vi "SiRealCenterFinder.vi"() -> ()   [LabVIEW 2019]
uses:
  <vilib>/userDefined/High Color/IMAQdx.ctl
panel:
  in  "AdjustCamera":T1={"+Y"=FALSE, "-Z"=FALSE, "Done"=FALSE, "+Z"=FALSE, "-Y"=FALSE, "-X"=FALSE, "+X"=FALSE, "MoveXYBy(mm)"=0.25, "Gcode"="", "MoveZBy(mm)"=0.1} {"MoveZBy(mm)" format="%#_13g"}
  out "CameraGcode":string
  in  "SiOnBPFiducials":path=path "C:/Users/TTUHEP/Documents/LabVIEW/Data/AssemblyIO_logs/Si2Fiducials_onBP.txt"
  out "Dev":dbl
  out "ImageCurrent":T2(plugin-control)
  out "Image2":T2(plugin-control)
  out "Image1":T2(plugin-control)
  out "Output XYZU":string
  in  "HexaboardEdges":path=path "C:/Users/TTUHEP/Documents/LabVIEW/Data/AssemblyIO_logs/PCB1_4Points.txt"
  in  "SiFiducials":path=path "C:/Users/TTUHEP/Documents/LabVIEW/Data/AssemblyIO_logs/Si2Fiducials.txt"
  in  "Component":enum16{"Baseplate", "Si", "SiOnBP", "PCB"}(ring)=enum."Si"
  in  "BasePlateEdges":path=path "C:/Users/TTUHEP/Documents/LabVIEW/Data/AssemblyIO_logs/Baseplate1CuPoints.txt"
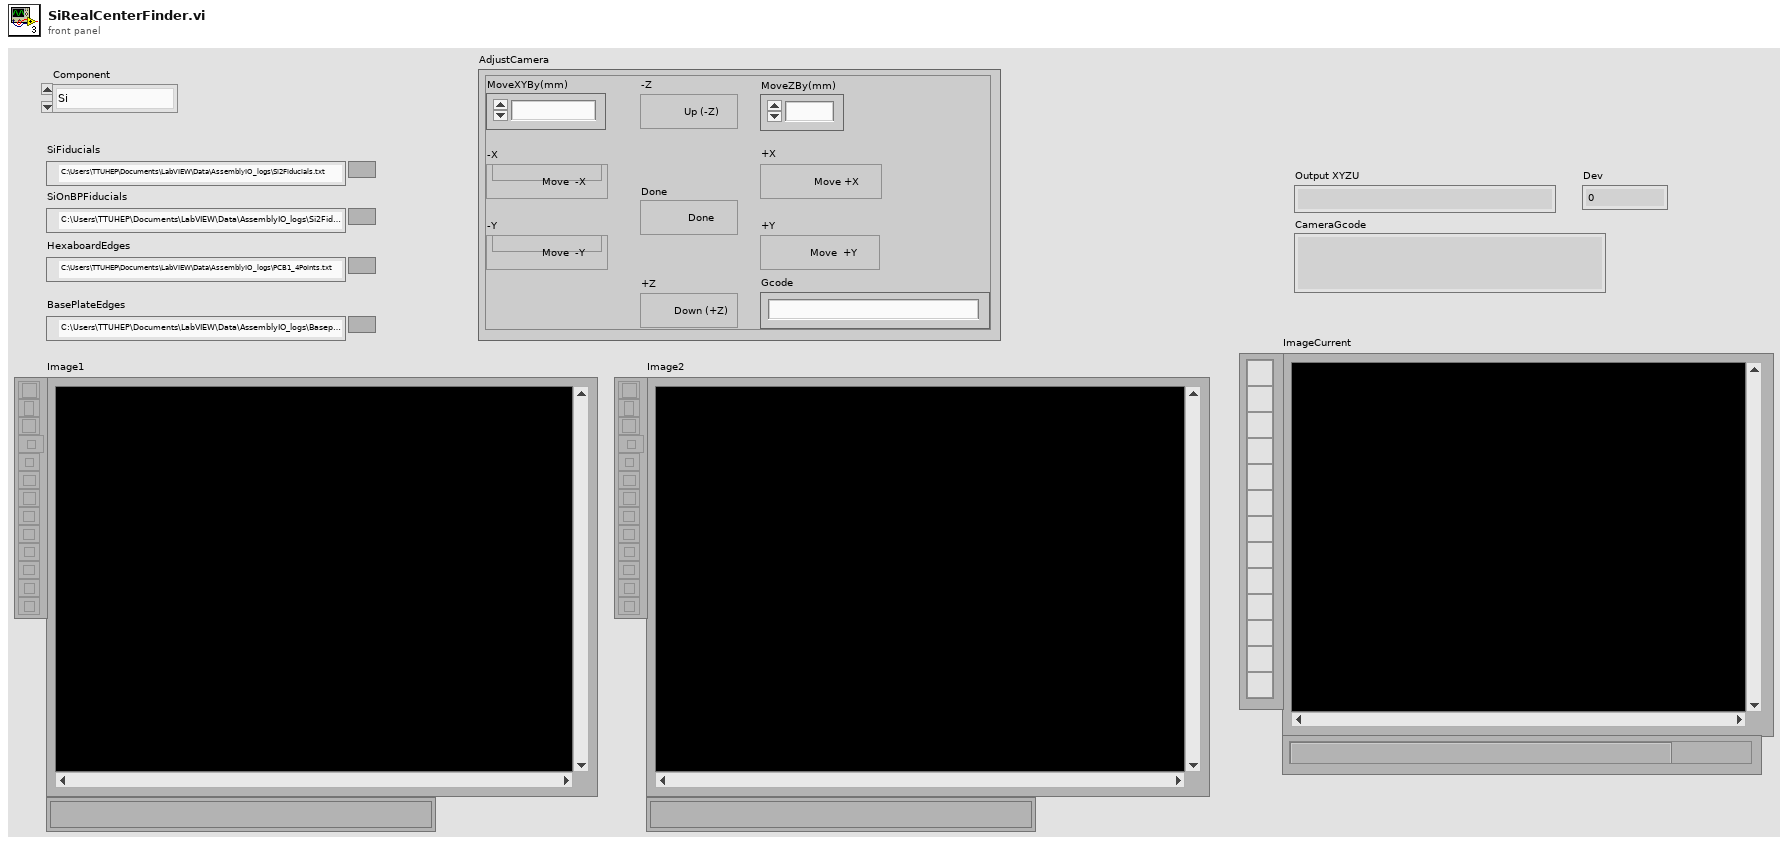
[diagram p1: front panel]
types:
  T1 = cluster{"+Y":bool, "-Z":bool, "Done":bool, "+Z":bool, "-Y":bool, "-X":bool, "+X":bool, "MoveXYBy(mm)":dbl, "Gcode":string, "MoveZBy(mm)":dbl}
  T2 = typedef "IMAQ Image.ctl" = refnum<image>
  T3 = typedef "IMAQdx.ctl" = refnum<k21>
  T4 = typedef "Image Type" = u32
  T5 = cluster{"Position":cluster{"X":sgl, "Y":sgl}, "Radius":dbl, "Score":dbl}
  T6 = enum16{"Left Button", "Center Button", "Right Button", "Window Close"}
  T7 = enum16{"open", "replace", "create", "open or create", "replace or create", "replace or create with confirmation"}
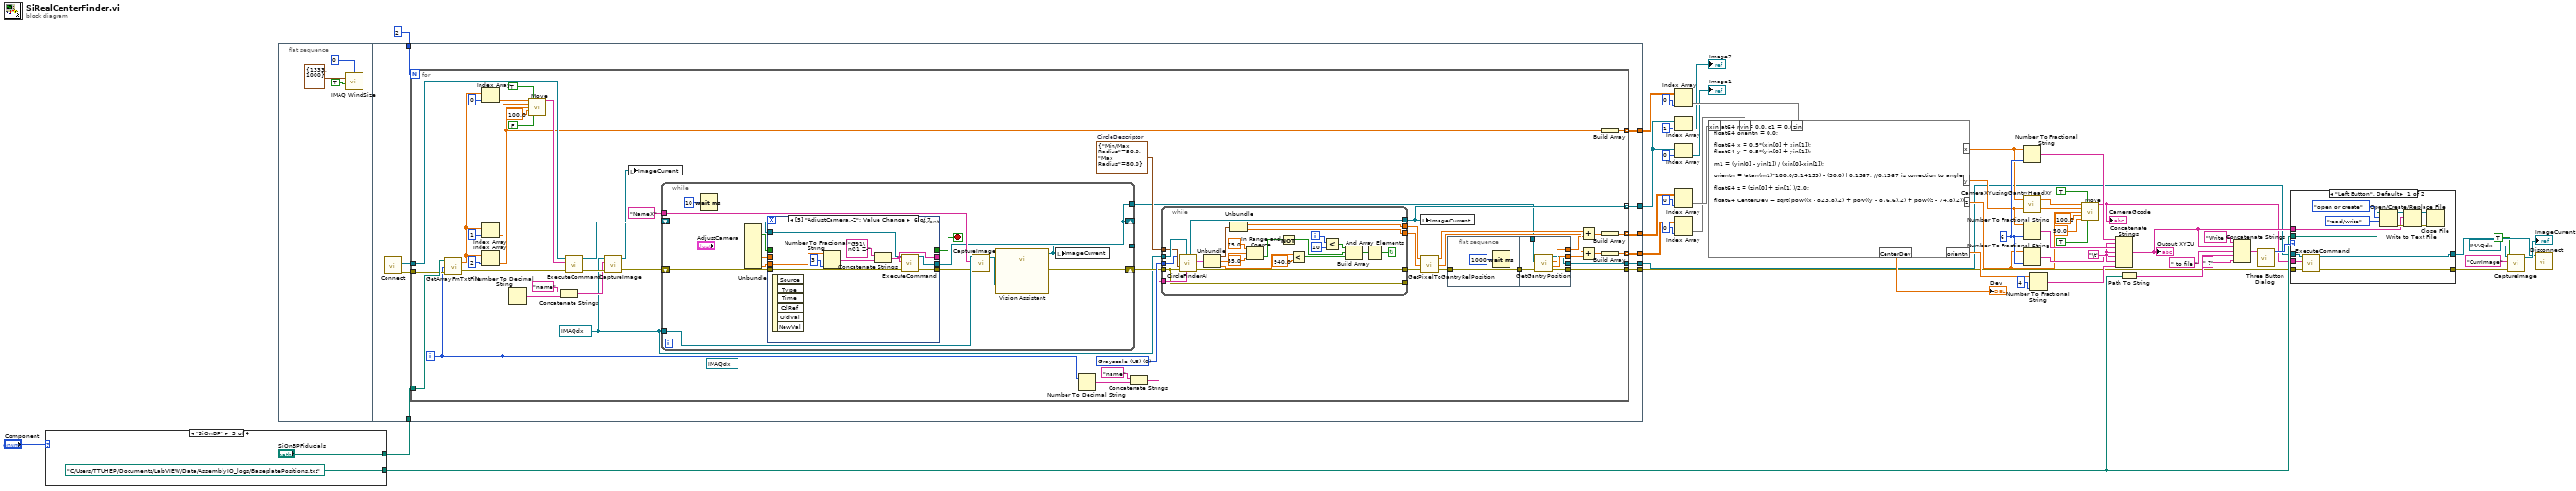
[diagram p0: block diagram]
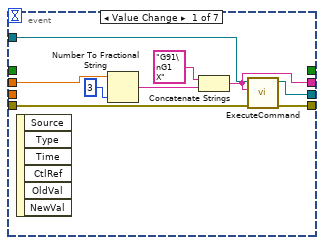
[diagram p3: hidden frame]
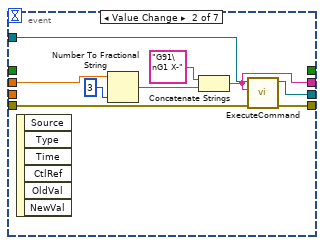
[diagram p4: hidden frame]
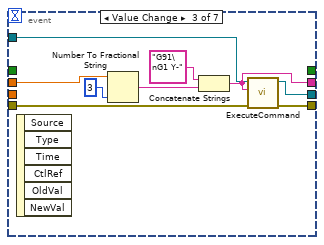
[diagram p5: hidden frame]
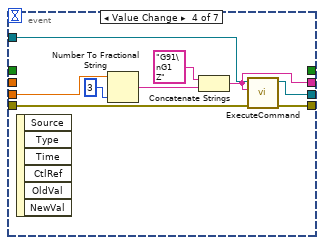
[diagram p6: hidden frame]
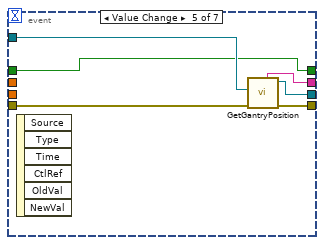
[diagram p7: hidden frame]
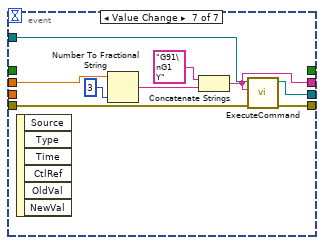
[diagram p8: hidden frame]
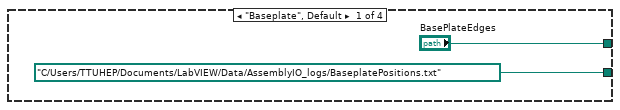
[diagram p9: hidden frame]
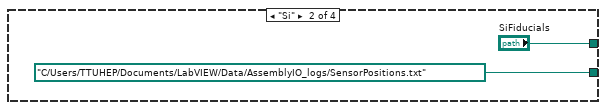
[diagram p10: hidden frame]
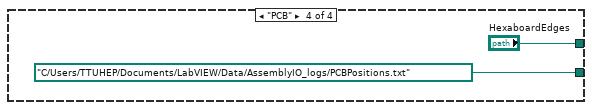
[diagram p11: hidden frame]
diagram:
  w49 = "\t"
  w46 = i16 6 ("width (-)")
  n1 = case shown="\"SiOnBP\"" "Component" {
    tunnel: ["BasePlateEdges" "SiFiducials" "SiOnBPFiducials" "HexaboardEdges"] -> w52
    tunnel: [path "C:/Users/TTUHEP/Documents/LabVIEW/Data/AssemblyIO_logs/BaseplatePositions.txt" ("OutFile") path "C:/Users/TTUHEP/Documents/LabVIEW/Data/AssemblyIO_logs/SensorPositions.txt" ("OutFile") path "C:/Users/TTUHEP/Documents/LabVIEW/Data/AssemblyIO_logs/BaseplatePositions.txt" ("OutFile") path "C:/Users/TTUHEP/Documents/LabVIEW/Data/AssemblyIO_logs/PCBPositions.txt" ("OutFile")] -> w37
    frame "Baseplate", Default {
    }
    frame "Si" {
    }
    frame "SiOnBP" {
    }
    frame "PCB" {
    }
  }
  n2 = flat-sequence {
    tunnel: 2 -> [w74]
    tunnel: w52 -> [w73]
    tunnel: [w72] -> w6
    tunnel: [w71] -> w5
    tunnel: [w68] -> w17
    tunnel: [w67] -> w35
    tunnel: [w66] -> w31
    tunnel: [w65] -> w33
    frame #0 {
      n3 = call "IMAQ WindSize"("Scrollbars? (N)"=TRUE, "Width & Height"=cluster{"Width":i32, "Height":i32} {"Width"=1333, "Height"=1000}, "Window Number"=0) -> ()  [unwired: 3 in, 3 out]
    }
    frame #1 {
      n4 = call "Connect.vi"() -> ("error out"=w70:errorcluster, "controller"=w69:refnum<k24>)  [unwired: 10 in]
      n5 = for {
        N: w74 -> [_]
        tunnel: w73 -> [w119]
        tunnel: w69 -> [w114]
        tunnel: w70 -> [w113]
        tunnel: [w88] -> w72
        tunnel: [w85] -> w71
        tunnel: [w93] -> w68 mode=indexing
        tunnel: [w109] -> w67 mode=indexing
        tunnel: [w107] -> w66 mode=indexing
        tunnel: [w106] -> w65 mode=indexing
        i -> [w78]
        (unwired) T3 "cam0" ("Camera")
        w98 = cluster{"Min/Max Radius":dbl, "Max Radius":dbl} {"Min/Max Radius"=50.0, "Max Radius"=80.0}  # CircleDescriptor
        w76 = T3 "cam0" ("Session In")
        w97 = T4 0 items=["Grayscale (U8)", "Grayscale (I16)", "Grayscale (SGL)", "Complex (CSG)", "RGB (U32)", "HSL (U32)", "RGB (U64)", "Grayscale (U16)"] ("Image Type")
        n6 = call "GetArrayFmTxtFile.vi"("error in"=w113, "LineNo."=w78, "TextFile"=w119) -> ("error out"=w112:errorcluster, "Array"=w120:dbl[])
        n7 = Index Array(array=w120, index=0) -> (element=w104:dbl)
        n8 = Index Array(array=w120, index=1) -> (element=w102:dbl)
        n9 = Index Array(array=w120, index=2) -> (element=w108:dbl)
        n10 = Number To Decimal String(number=w78) -> (decimal integer string=w80:string)  [unwired: 1 in]
        n11 = call "Move.vi"("X"=w104, "Absolute"=TRUE, "Y"=w102, "Z"=w108, "SpeedXY (mm/s)"=100.0, "Move Z first"=FALSE) -> ("Position Gcode"=w115:string)  [unwired: 9 in]
        n12 = Concatenate Strings("name" ("string"), w80) -> (w77:string)
        n13 = call "ExecuteCommand.vi"("error in (no error)"=w112, "Command Code"=w115, "controller in"=w114) -> ("error out"=w82:errorcluster, "controller out"=w91:refnum<k24>)  [unwired: 6 in, 1 out]
        n14 = call "CaptureImage.vi"("Camera"=w76, "ImageName"=w77, "error in (no error)"=w82) -> ("Image"=w75:T2, "error out"=w81:errorcluster)  [unwired: 4 in]
        n15 = local write "ImageCurrent"(w75) -> ()
        n16 = while {
          shift-right: [w140] -> w90
          shift-left: w81 -> [w147]
          shift-right: [w137] -> _
          shift-left: w91 -> [w146]
          tunnel: "NameX" ("ImageName") -> [w142]
          tunnel: w76 -> [w143]
          tunnel: [w136] -> _
          tunnel: [w137] -> w89
          stop <- w145 stop-if-true
          n17 = Wait (ms)(milliseconds to wait=u32 10) -> ()  [unwired: 1 out]
          n18 = Unbundle("AdjustCamera") -> ("Done"=w132:bool, "MoveXYBy(mm)"=w134:dbl, "MoveZBy(mm)"=w133:dbl)  [unwired: 7 out]
          n19 = event shown="[5] \"AdjustCamera.-Z\": Value Change" {
            selector: _ -> [_ _ _ _ _ _ _]
            dyn-events: _ -> [_ _ _ _ _ _ _]
            timeout: _ -> [_ _ _ _ _ _ _]
            tunnel: w134 -> [w153 w157 w166 _ _ _ w199]
            tunnel: w147 -> [w152 w161 w170 w179 w188 w194 w203]
            tunnel: [w151 w160 w169 w176 w186 w193 w202] -> w141
            tunnel: w146 -> [w150 w162 w171 w180 w189 w195 w204]
            tunnel: [w149 w159 w168 w177 w187 w192 w201] -> w137
            tunnel: [w148 w158 w167 w178 w184 w191 w200] -> _
            tunnel: [_ _ _ _ w185 _ _] -> w145
            tunnel: w133 -> [_ _ _ w175 _ w190 _]
            tunnel: w132 -> [_ _ _ _ w185 _ _]
            event "AdjustCamera.+X": Value Change {
              n20 = event-data() -> ()  [unwired: 1 in, 6 out]
              n21 = Number To Fractional String(number=w153, precision (6)=3) -> (F-format string=w156:string)  [unwired: 2 in]
              n22 = Concatenate Strings("G91\nG1 X", w156) -> (w148:string)
              n23 = call "ExecuteCommand.vi"("error in (no error)"=w152, "Command Code"=w148, "controller in"=w150) -> ("error out"=w151:errorcluster, "controller out"=w149:refnum<k24>)  [unwired: 6 in, 1 out]
            }
            event "AdjustCamera.-X": Value Change {
              n24 = event-data() -> ()  [unwired: 1 in, 6 out]
              n25 = Number To Fractional String(number=w157, precision (6)=3) -> (F-format string=w165:string)  [unwired: 2 in]
              n26 = Concatenate Strings("G91\nG1 X-", w165) -> (w158:string)
              n27 = call "ExecuteCommand.vi"("error in (no error)"=w161, "Command Code"=w158, "controller in"=w162) -> ("error out"=w160:errorcluster, "controller out"=w159:refnum<k24>)  [unwired: 6 in, 1 out]
            }
            event "AdjustCamera.-Y": Value Change {
              n28 = event-data() -> ()  [unwired: 1 in, 6 out]
              n29 = Number To Fractional String(number=w166, precision (6)=3) -> (F-format string=w174:string)  [unwired: 2 in]
              n30 = Concatenate Strings("G91\nG1 Y-", w174) -> (w167:string)
              n31 = call "ExecuteCommand.vi"("error in (no error)"=w170, "Command Code"=w167, "controller in"=w171) -> ("error out"=w169:errorcluster, "controller out"=w168:refnum<k24>)  [unwired: 6 in, 1 out]
            }
            event "AdjustCamera.+Z": Value Change {
              n32 = event-data() -> ()  [unwired: 1 in, 6 out]
              n33 = Number To Fractional String(number=w175, precision (6)=3) -> (F-format string=w183:string)  [unwired: 2 in]
              n34 = Concatenate Strings("G91\nG1 Z", w183) -> (w178:string)
              n35 = call "ExecuteCommand.vi"("error in (no error)"=w179, "Command Code"=w178, "controller in"=w180) -> ("error out"=w176:errorcluster, "controller out"=w177:refnum<k24>)  [unwired: 6 in, 1 out]
            }
            event "AdjustCamera.Done": Value Change {
              n36 = event-data() -> ()  [unwired: 1 in, 6 out]
              n37 = call "GetGantryPosition.vi"("error in (no error)"=w188, "Controller In"=w189) -> ("error out"=w186:errorcluster, "controller out"=w187:refnum<k24>, "Position_XYZ"=w184:string)  [unwired: 3 in, 4 out]
            }
            event "AdjustCamera.-Z": Value Change {
              n38 = event-data() -> ()  [unwired: 1 in, 6 out]
              n39 = Number To Fractional String(number=w190, precision (6)=3) -> (F-format string=w198:string)  [unwired: 2 in]
              n40 = Concatenate Strings("G91\nG1 Z-", w198) -> (w191:string)
              n41 = call "ExecuteCommand.vi"("error in (no error)"=w194, "Command Code"=w191, "controller in"=w195) -> ("error out"=w193:errorcluster, "controller out"=w192:refnum<k24>)  [unwired: 6 in, 1 out]
            }
            event "AdjustCamera.+Y": Value Change {
              n42 = event-data() -> ()  [unwired: 1 in, 6 out]
              n43 = Number To Fractional String(number=w199, precision (6)=3) -> (F-format string=w207:string)  [unwired: 2 in]
              n44 = Concatenate Strings("G91\nG1 Y", w207) -> (w200:string)
              n45 = call "ExecuteCommand.vi"("error in (no error)"=w203, "Command Code"=w200, "controller in"=w204) -> ("error out"=w202:errorcluster, "controller out"=w201:refnum<k24>)  [unwired: 6 in, 1 out]
            }
          }
          n46 = call "CaptureImage.vi"("Camera"=w143, "ImageName"=w142, "error in (no error)"=w141) -> ("Image"=w139:T2, "error out"=w138:errorcluster)  [unwired: 4 in]
          n47 = call "Vision Assistant"("Image In"=w139, "error in"=w138) -> ("Image Out"=w136:T2, "error out"=w140:errorcluster)  [unwired: 24 in]
          n48 = local write "ImageCurrent"(w136) -> ()
        }
        n49 = Number To Decimal String(number=w78) -> (decimal integer string=w111:string)  [unwired: 1 in]
        n50 = Concatenate Strings("name" ("string"), w111) -> (w99:string)
        n51 = while {
          tunnel: w99 -> [w229]
          tunnel: w76 -> [w228]
          tunnel: [w208] -> _
          tunnel: w98 -> [w227]
          tunnel: w97 -> [w226]
          tunnel: [w225] -> w96
          tunnel: [w224] -> w93
          tunnel: [w210] -> w95
          tunnel: [w209] -> w94
          tunnel: w90 -> [w208]
          i -> [w231]
          stop <- w211 continue-if-true
          n52 = call "CircleFinderAI.vi"("Image Name"=w229, "Session In"=w228, "error in (no error)"=w208, "Circle Descriptor"=w227, "Image Type"=w226) -> ("error out"=w225:errorcluster, "Circle0"=w223:T5, "Image"=w224:T2)  [unwired: 2 in, 2 out]
          n53 = Unbundle(w223) -> ("Position"=w217:cluster{"X":sgl, "Y":sgl}, "Radius"=w218:dbl, "Score"=w222:dbl)
          n54 = Unbundle(w217) -> ("X"=w210:sgl, "Y"=w209:sgl)
          n55 = In Range and Coerce(upper limit=75.0, x=w218, lower limit=55.0) -> (In Range?=w216:bool)  [unwired: 1 out]
          n56 = Not(x=w216) -> (.not. x?=w214:bool)
          n57 = Less?(x=w222, y=940.0) -> (x < y?=w213:bool)
          n58 = Less?(x=w231, y=10) -> (x < y?=w215:bool)
          n59 = Build Array(w215, w214, w213) -> (w212:bool[])
          n60 = And Array Elements(Boolean array=w212) -> (logical AND=w211:bool)
        }
        n61 = local write "ImageCurrent"(w93) -> ()
        n62 = call "GetPixelToGantryRelPosition.vi"("error in (no error)"=w96, "PixelY"=w94, "PixelX"=w95) -> ("error out"=w83:errorcluster, "YmmRelGH"=w101:dbl, "XmmRelGH"=w105:dbl)
        n63 = flat-sequence {
          tunnel: [w124] -> w84
          tunnel: w83 -> [w124]
          tunnel: w89 -> [w131]
          tunnel: [w130] -> w88
          tunnel: [w129] -> w87
          tunnel: [w128] -> w86
          tunnel: [w127] -> w85
          tunnel: w84 -> [w126]
          frame #0 {
            n64 = Wait (ms)(milliseconds to wait=u32 1000) -> ()  [unwired: 1 out]
          }
          frame #1 {
            n65 = call "GetGantryPosition.vi"("error in (no error)"=w126, "Controller In"=w131) -> ("error out"=w130:errorcluster, "Position Y"=w129:dbl, "Position X"=w128:dbl, "controller out"=w127:refnum<k24>)  [unwired: 3 in, 3 out]
          }
        }
        n66 = Add(x=w105, y=w86) -> (x+y=w103:dbl)
        n67 = Add(x=w101, y=w87) -> (x+y=w100:dbl)
        n68 = Build Array(w108) -> (w109:dbl[])
        n69 = Build Array(w103) -> (w106:dbl[])
        n70 = Build Array(w100) -> (w107:dbl[])
      }
    }
  }
  n71 = Index Array(array=w35, index (col)=0 ("disabled index (col)")) -> (element=w23:dbl[])  [unwired: 1 in]
  n72 = Index Array(array=w17, index=1 ("length")) -> (element=→"Image2":T2)
  n73 = Index Array(array=w17, index=0 ("length")) -> (element=→"Image1":T2)
  n74 = Index Array(array=w33, index (col)=0 ("disabled index (col)")) -> (element=w25:dbl[])  [unwired: 1 in]
  n75 = Index Array(array=w31, index (col)=0 ("disabled index (col)")) -> (element=w24:dbl[])  [unwired: 1 in]
  n76 = formula code="float64 m1 = 0.0, c1 = 0.0;\nfloat64 orientn = 0.0;\n\nfloat64 x = 0.5*(xin[0] + xin[1]); \nfloat64 y = 0.5*(yin[0] + yin[1]);\n\nm1 = (yin[0] - yin[1]) / (xin[0]-xin[1]);\n\norientn = (atan(m1)*180.0/3.14159) - (30.0)+0.1567; //0.1567 is correction to angle\n\nfloat64 z = (zin[0] + zin[1] )/2.0;\n\nfloat64 CenterDev = sqrt( pow((x - 823.8),2) + pow((y - 876.6),2) + pow((z - 74.8),2));"("xin"=w25, "yin"=w24, "zin"=w23) -> ("orientn"=w22:dbl, "x"=w11:dbl, "y"=w8:dbl, "z"=w7:dbl, "CenterDev"=→"Dev":dbl)
  n77 = Number To Fractional String(number=w11, precision (6)=w46) -> (F-format string=w51:string)  [unwired: 2 in]
  n78 = call "CameraXYusingGantryHeadXY.vi"("GantryY"=w8, "GantryX"=w11) -> ("CamY"=w9:dbl, "CamX"=w10:dbl)
  n79 = Number To Fractional String(number=w8, precision (6)=w46) -> (F-format string=w50:string)  [unwired: 2 in]
  n80 = Number To Fractional String(number=w7, precision (6)=w46) -> (F-format string=w45:string)  [unwired: 2 in]
  n81 = Number To Fractional String(number=w22, precision (6)=i16 4 ("width (-)")) -> (F-format string=w47:string)  [unwired: 2 in]
  n82 = call "Move.vi"("X"=w10, "Absolute"=TRUE, "Y"=w9, "Z"=w7, "SpeedXY (mm/s)"=100.0, "SpeedZ (mm/s)"=50.0, "Move Z first"=TRUE) -> ("Position Gcode"=w2:string)  [unwired: 8 in]
  "CameraGcode" <- w2
  n83 = Concatenate Strings(w51, w49, w50, w49, w45, w49, w47) -> (w43:string)
  "Output XYZU" <- w43
  n84 = Path To String(path=w37) -> (string=w41:string)
  n85 = Concatenate Strings("Write ", w43, " to file ", w41, " ?" ("string")) -> (w39:string)
  n86 = call <vilib>:"Three Button Dialog.vi"("message"=w39) -> ("Which Button?"=w38:T6)  [unwired: 10 in]
  n87 = case shown="\"Left Button\", Default" w38 {
    tunnel: w43 -> [w238 _]
    tunnel: w37 -> [w237 _]
    tunnel: w6 -> [w236 w245]
    tunnel: w2 -> [w235 _]
    tunnel: w5 -> [w234 w246]
    tunnel: [w233 w245] -> w4
    tunnel: [w232 w246] -> w3
    frame "Left Button", Default {
      n88 = call "ExecuteCommand.vi"("error in (no error)"=w236, "Command Code"=w235, "controller in"=w234) -> ("error out"=w233:errorcluster, "controller out"=w232:refnum<k24>)  [unwired: 6 in, 1 out]
      n89 = Open/Create/Replace File(file path (use dialog)=w237, operation (0:open)=T7."open or create", access (0:read/write)=enum16{"read/write", "read-only", "write-only"}."read/write") -> (refnum out=w244:refnum<file>, error out=w241:errorcluster)  [unwired: 3 in, 1 out]
      n90 = Write to Text File(file (use dialog)=w244, text=w238, error in=w241) -> (refnum out=w239:refnum<file>, error out=w240:errorcluster)  [unwired: 1 in, 1 out]
      n91 = Close File(refnum=w239, error in=w240) -> ()  [unwired: 2 out]
    }
    frame "Center Button" {
    }
  }
  n92 = call "CaptureImage.vi"("Camera"=T3 "cam0", "ImageName"="CurrImage", "Draw50MicroCircleAtCenter"=TRUE, "error in (no error)"=w4) -> ("Image"=→"ImageCurrent":T2, "error out"=w16:errorcluster)  [unwired: 3 in]
  n93 = call "Disconnect.vi"("error in (no error)"=w16, "controller"=w3) -> ()  [unwired: 9 in, 1 out]
